vi "INI_RS232_RFID.vi"(0 "Device INI Config File Path":path=path "D:/LABVIEW/Examples/INI Devices/DeviceConfig.ini", 2 "MListBox Row":u16=2 max=8, 7 "MCListbox Ref":refnum<vi>) -> (5 "RFID Power":u16, 6 "COM Port":refnum<visa-resource-name>, 8 "Dev OK":bool, 9 "Handle":u32, 10 "error out":errorcluster)   [LabVIEW 2018]
uses:
  <vilib>/Utility/miscctls.llb/LVRowAndColumnTypeDef.ctl
  <vilib>/Utility/config.llb/Read Key (String).vi
  <vilib>/Utility/config.llb/Read Key (I32).vi
  <vilib>/Utility/config.llb/NI_LVConfig.lvlib
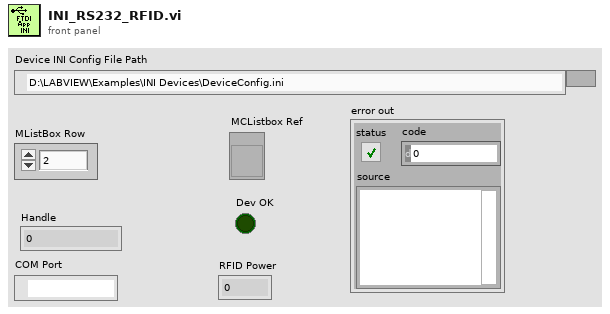
[diagram p1: front panel]
types:
  T1 = typedef "LVRowAndColumnTypeDef.ctl" = cluster{"Row":i32, "Column":i32}
  T2 = typedef "NI_LVConfig.lvlib/Config Data RefNum.ctl" = refnum<k1>
  T3 = cluster{"Type":u32, "VID":string, "PID":string, "Serial Number":string, "Description":string}
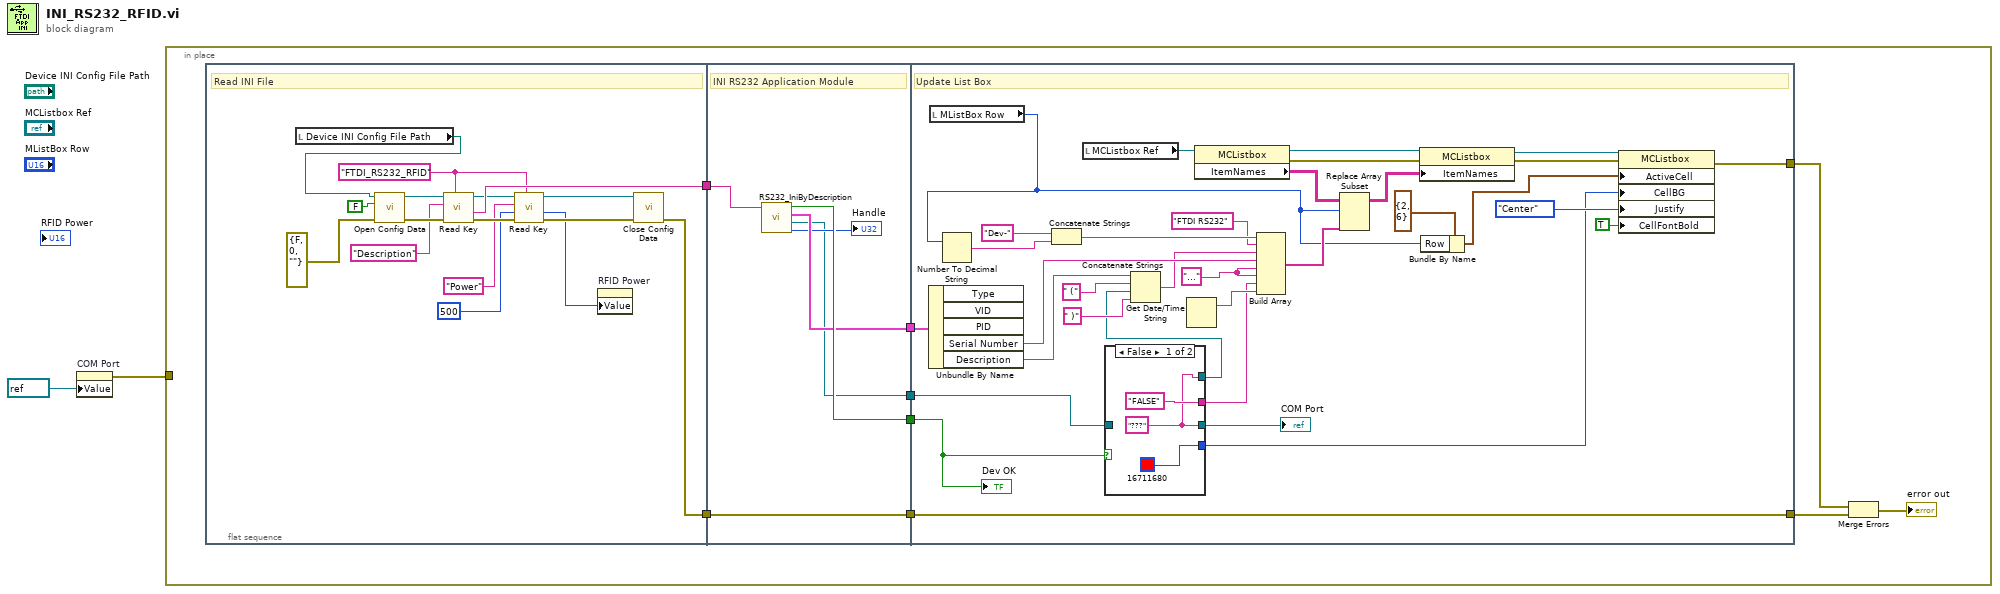
[diagram p0: block diagram]
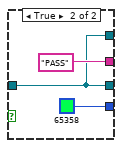
[diagram p2: hidden frame]
diagram:
  n1 = property on="COM Port" class="VISAName"("Value"=refnum<visa-resource-name> "???" ("COM Port")) -> (error out=w2:errorcluster)  [unwired: 2 in, 1 out]
  n2 = in-place {
    in-place-border: w2 -> [_]
    n3 = flat-sequence {
      tunnel: [w21] -> w11
      tunnel: [w20] -> w6
      tunnel: w11 -> [w33]
      tunnel: [w33] -> w9
      tunnel: w6 -> [w32]
      tunnel: [w31] -> w5
      tunnel: [w30] -> w4
      tunnel: [w28] -> w3
      tunnel: [w53] -> w10
      tunnel: [w52] -> w8
      tunnel: w9 -> [w52]
      tunnel: w5 -> [w41]
      tunnel: w4 -> [w44]
      tunnel: w3 -> [w36]
      frame #0 {
        w15 = "FTDI_RS232_RFID" ("section")
        # "Read INI File"
        n4 = local read "Device INI Config File Path"() -> (w23:path)
        n5 = call <vilib>:"Open Config Data.vi"("error in (no error)"=errorcluster {"status"=FALSE, "code"=0, "source"=""} ("error constant"), "create file if necessary (T)"=FALSE, "configuration file path"=w23) -> ("error out"=w25:errorcluster, "refnum"=w26:T2)  [unwired: 6 in, 1 out]
        n6 = call-poly <vilib>:"Read Key.vi"("section"=w15, "error in (no error)"=w25, "key"="Description", "refnum"=w26) -> ("error out"=w18:errorcluster, "value"=w20:string, "refnum out"=w19:T2)  [unwired: 4 in, 1 out]
        n7 = call-poly <vilib>:"Read Key.vi"("section"=w15, "error in (no error)"=w18, "default value"=500, "key"="Power", "refnum"=w19) -> ("error out"=w16:errorcluster, "value"=w12:i32, "refnum out"=w17:T2)  [unwired: 3 in, 1 out]
        n8 = property on="RFID Power" class="DigNum (strict)"("Value"=w12) -> ()  [unwired: 2 in, 2 out]
        n9 = call <vilib>:"Close Config Data.vi"("error in (no error)"=w16, "refnum"=w17) -> ("error out"=w21:errorcluster)  [unwired: 8 in, 1 out]
      }
      frame #1 {
        # "INI RS232 Application Module"
        n10 = call "RS232_IniByDescription.vi"("Description"=w32) -> ("Handle"=→"Handle":u32, "COM Port"=w28:refnum<visa-resource-name>, "Device Information"=w30:T3, "Ok?"=w31:bool)  [unwired: 7 in]
      }
      frame #2 {
        w42 = "..."
        # "Update List Box"
        n11 = Unbundle By Name(w44) -> ("Serial Number"=w43:string, "Description"=w40:string)  [unwired: 3 out]
        n12 = local read "MListBox Row"() -> (w46:u16)
        n13 = Number To Decimal String(number=w46) -> (decimal integer string=w49:string)  [unwired: 1 in]
        n14 = Concatenate Strings("Dev-", w49) -> (w48:string)
        n15 = local read "MCListbox Ref"() -> (w47:refnum<vi>)
        n16 = case shown="False" w41 {
          tunnel: [u32 16711680 u32 65358] -> w55
          tunnel: ["FALSE" ("element") "PASS" ("element")] -> w54
          tunnel: w36 -> [_ w70]
          tunnel: [w67 w70] -> w35
          tunnel: [w67 w70] -> w34
          frame False {
            w67 = "???"
          }
          frame True {
          }
        }
        "COM Port" <- w35
        n17 = Concatenate Strings(w40, " (", w34, " )") -> (w39:string)
        n18 = Get Date/Time String() -> (date string=w58:string)  [unwired: 3 in, 1 out]
        n19 = property class="MCListbox"(reference=w47) -> (reference out=w60:refnum<vi>, error out=w61:errorcluster, "ItemNames"=w62:string[][])  [unwired: 1 in]
        n20 = Build Array(w48, "FTDI RS232", w39, w43, w42, w42, w54, w58) -> (w64:string[])
        n21 = Replace Array Subset(array=w62, new element=w64, index (row)=w46) -> (w63:string[][])  [unwired: 1 in]
        n22 = property class="MCListbox"(reference=w60, error in=w61, "ItemNames"=w63) -> (reference out=w65:refnum<vi>, error out=w66:errorcluster)
        n23 = Bundle By Name(cluster=T1 {"Row"=2, "Column"=6} ("Active Cell:Active Cell"), "Row"=w46) -> (w56:T1)
        n24 = property class="MCListbox"(reference=w65, error in=w66, "ActiveCell"=w56, "CellBG"=w55, "Justify"=enum16{"Left", "Center", "Right"}."Center" ("Active Cell:Cell Justification"), "CellFontBold"=TRUE ("Active Cell:Cell Font:Bold")) -> (error out=w53:errorcluster)  [unwired: 1 out]
        "Dev OK" <- w41
      }
    }
    n25 = Merge Errors(w10, w8) -> (→"error out":errorcluster)
  }
